vi "Resolve D.vi"(10 "双字索引":dbl[](array[numeric]), 11 "字符串":string) -> (1 "有符号数据":dbl[](array[numeric]), 2 "解析双字数据":dbl[](array[numeric]) format="%#.6f", 3 "解析后的数据":i32[](array[numeric]))   [LabVIEW 2017]
panel:
  out "数字":i32[](array[numeric])
  out "数组 2":i32[](array[numeric])
  out "数组":string[](array[string])
  # "双字索引两数之间最小相差最好为2"
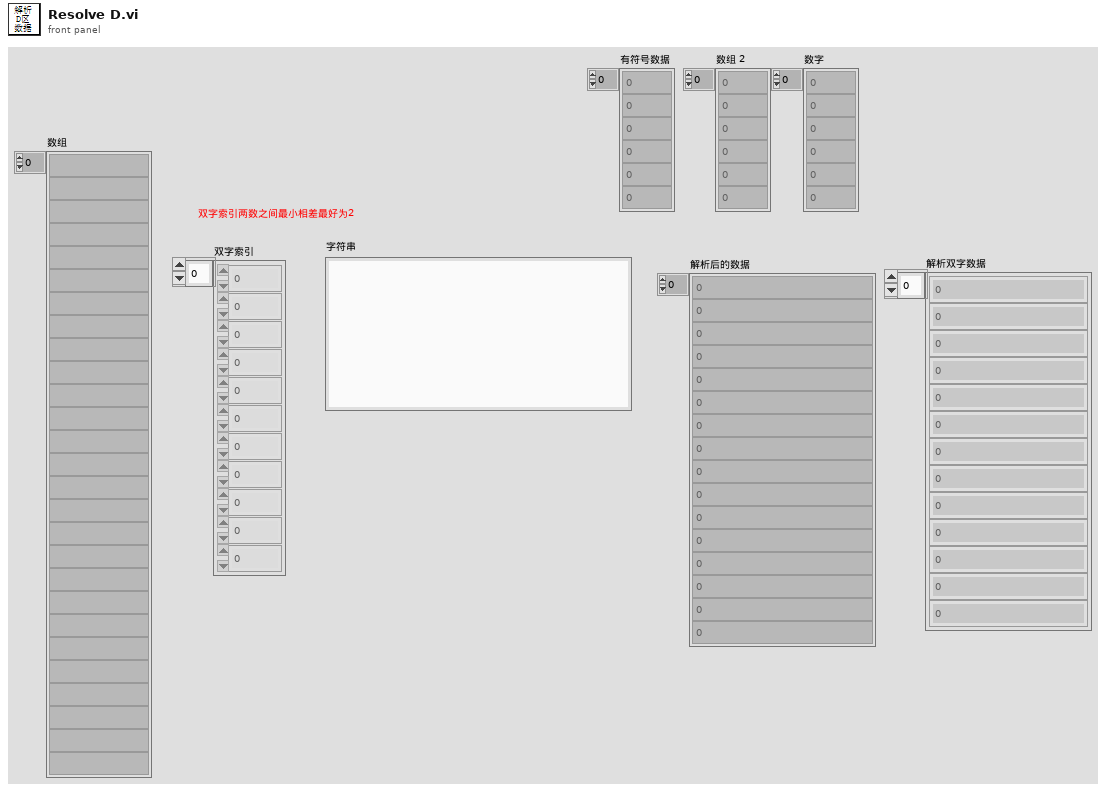
[diagram p1: front panel]
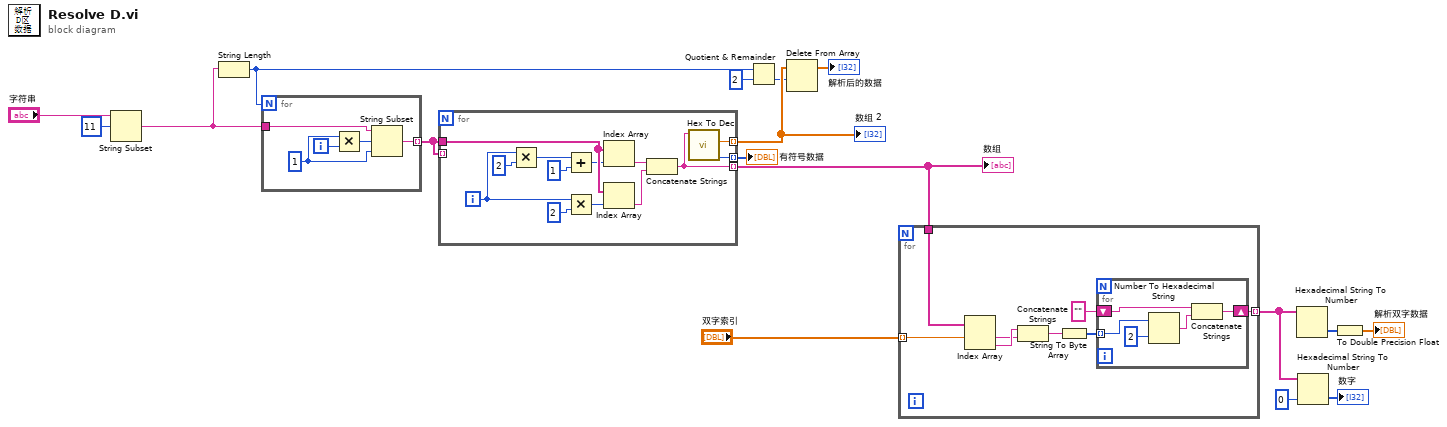
[diagram p0: block diagram]
diagram:
  n1 = String Subset(string="字符串", offset (0)=11 ("偏移量(0)")) -> (substring=w2:string)  [unwired: 1 in]
  n2 = String Length(string=w2) -> (length=w14:i32)
  n3 = for {
    N: w14 -> [_]
    tunnel: w2 -> [w22]
    tunnel: [w18] -> w17 mode=indexing
    i -> [w21]
    w20 = 1 ("长度（剩余）")
    n4 = Multiply(x=w20, y=w21) -> (x*y=w19:i32)
    n5 = String Subset(string=w22, offset (0)=w19, length (rest)=w20) -> (substring=w18:string)
  }
  n6 = for {
    tunnel: w17 -> [w29]
    tunnel: w17 -> [_] mode=indexing
    tunnel: [w25] -> w16 mode=indexing
    tunnel: [w24] -> w11 mode=indexing
    tunnel: [w23] -> w7 mode=indexing
    i -> [w33]
    n7 = Multiply(x=w33, y=2) -> (x*y=w32:i32)
    n8 = Add(x=w32, y=1) -> (x+y=w28:i32)
    n9 = Multiply(x=w33, y=2) -> (x*y=w30:i32)
    n10 = Index Array(array=w29, index=w28) -> (element=w27:string)
    n11 = Index Array(array=w29, index=w30) -> (element=w26:string)
    n12 = Concatenate Strings(w27, w26) -> (w24:string)
    n13 = call "Hex To Dec.vi"("十六进制字符串"=w24) -> ("32位整型"=w23:i32, "十进制整数"=w25:dbl)  [unwired: 7 in, 2 out]
  }
  "数组" <- w11
  "有符号数据" <- w7
  "数组 2" <- w16
  n14 = Quotient & Remainder(x=w14, y=2) -> (floor(x/y)=w12:i32)  [unwired: 1 out]
  n15 = Delete From Array(array=w16, length=w12) -> (array with subset deleted=→"解析后的数据":dbl[])  [unwired: 1 in, 1 out]
  n16 = for {
    tunnel: w11 -> [w43]
    tunnel: [w38] -> w6 mode=indexing
    tunnel: "双字索引" -> [w36] mode=indexing
    n17 = Index Array(array=w43, index #1=w36) -> (element #1=w41:string, element #2=w42:string)  [unwired: 1 in]
    n18 = Concatenate Strings(w42, w41) -> (w37:string)
    n19 = String To Byte Array(string=w37) -> (unsigned byte array=w40:u8[])
    n20 = for {
      tunnel: w40 -> [w48] mode=indexing
      shift-right: [w47] -> w38
      shift-left: "" -> [w46]
      n21 = Number To Hexadecimal String(1:i16 2 ("宽度(-)"), 2:w48) -> (0:w45:string)
      n22 = Concatenate Strings(w46, w45) -> (w47:string)
    }
  }
  n23 = Hexadecimal String To Number(string=w6) -> (number=w10:u32[])  [unwired: 2 in, 1 out]
  n24 = Hexadecimal String To Number(string=w6, default (0uL)=0 ("默认(0 U32)")) -> (number=→"数字":i32[])  [unwired: 1 in, 1 out]
  n25 = To Double Precision Float(number=w10) -> (double precision float=→"解析双字数据":dbl[])
